vi "放入试件后吸声量A2计算.vi"(9 "频率":dbl[](array[numeric]), 10 "平均混响时间T2":dbl[](array[numeric])) -> (2 "混响室吸声量A2":dbl[](array[numeric]))   [LabVIEW 2020]
uses:
  setup/support/rev_setup.lvlib
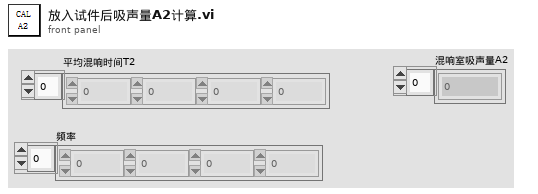
[diagram p1: front panel]
types:
  T1 = typedef "rev_setup.lvlib/EMdata.ctl" = cluster{"大气压力(kPa)":dbl, "大气压力(kPa) 2":dbl, "相对湿度(%)":dbl, "相对湿度(%)2":dbl, "大气温度(℃)":dbl, "大气温度(℃)2":dbl, "声速(m/s)":dbl, "声速(kPa)2":dbl, "混响室容积(立方米) ":dbl, "试件面积(平方米)，S":dbl, "分立吸声体个数，n":dbl}
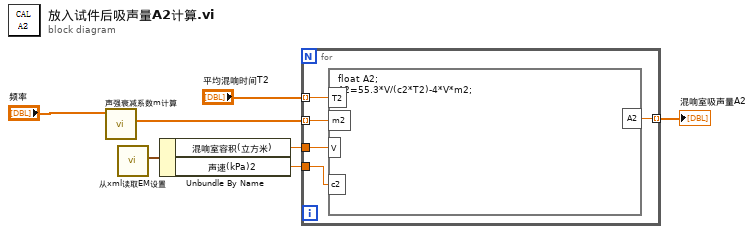
[diagram p0: block diagram]
diagram:
  n1 = call "声强衰减系数m计算.vi"("输入频率"="频率") -> ("声强衰减系数m2"=w1:dbl[])  [unwired: 9 in, 1 out]
  n2 = call "从xml读取EM设置.vi"() -> ("EM data"=w5:T1)  [unwired: 11 in]
  n3 = Unbundle By Name(w5) -> ("混响室容积(立方米)"=w4:dbl, "声速(kPa)2"=w3:dbl)
  n4 = for {
    tunnel: "平均混响时间T2" -> [w12] mode=indexing
    tunnel: w4 -> [w11]
    tunnel: w3 -> [w10]
    tunnel: [w9] -> w6 mode=indexing
    tunnel: w1 -> [w8] mode=indexing
    n5 = formula code="float A2;\nA2=55.3*V/(c2*T2)-4*V*m2;"("T2"=w12, "V"=w11, "c2"=w10, "m2"=w8) -> ("A2"=w9:dbl)
  }
  "混响室吸声量A2" <- w6
